vi "Get DDGIOC Period.vi"(8 "error in (no error)":errorcluster, 11 "period":cluster{}) -> (0 "error out":errorcluster, 2 "function return":u32, 3 "period out":cluster{})   [LabVIEW 2014, in "atmcd32d.lvlib"]
doc: "unsigned int WINAPI GetDDGIOCPeriod(at_u64 * period);"
uses:
  atmcd32d.lvlib
  atmcd32d.dll
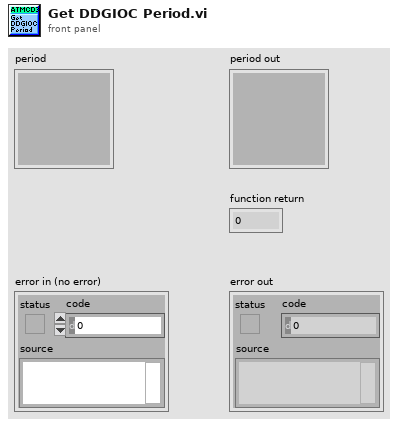
[diagram p1: front panel]
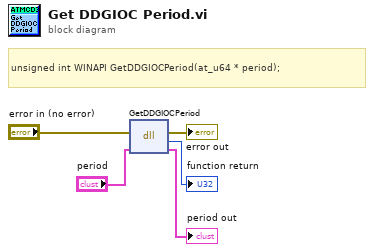
[diagram p0: block diagram]
diagram:
  # "unsigned int WINAPI GetDDGIOCPeriod(at_u64 * period);"
  n1 = dll-call lib="C:/Users/Bakir/Documents/Lambda2-Testing/lib/Andorlib/atmcd32d.*" fn="GetDDGIOCPeriod"(error in="error in (no error)", "period"="period") -> (error out=→"error out":errorcluster, →"function return":u32, "period"=→"period out":cluster{})  [unwired: 2 in, 1 out]
